vi "EventBuilder.ProcEvents.vi"(0 "i ref in":refnum<vi>, 5 "error in (no error)":errorcluster) -> (14 "i ref out":refnum<vi>, 19 "error out":errorcluster)   [LabVIEW 2014, in "EventBuilder.lvlib"]
doc: "This method is used to define the events the object will listen to. Add your own events here."
uses:
  EventBuilder.lvlib
  CSCore/BaseProcess/BaseProcess.event definition.ctl
  CSCore/CAEObj/CAEObj.event definition.ctl
  CSCore/BaseProcess/BaseProcess.descriptor string definition.ctl
  CSCore/BaseProcess/BaseProcess.lvlib
  CSCore/CAEObj/CAEObj.lvlib
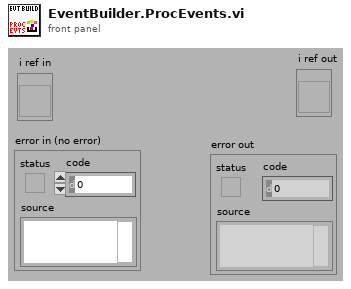
[diagram p1: front panel]
types:
  T1 = typedef "BaseProcess.lvlib/BaseProcess.event definition.ctl" = cluster{"CAEEvtDef":T2, "Data Descriptor":T3}
  T2 = typedef "CAEObj.lvlib/CAEObj.event definition.ctl" = cluster{"URL":string, "enable":bool, "ignoreResID":bool}
  T3 = typedef "BaseProcess.lvlib/BaseProcess.descriptor string definition.ctl" = string
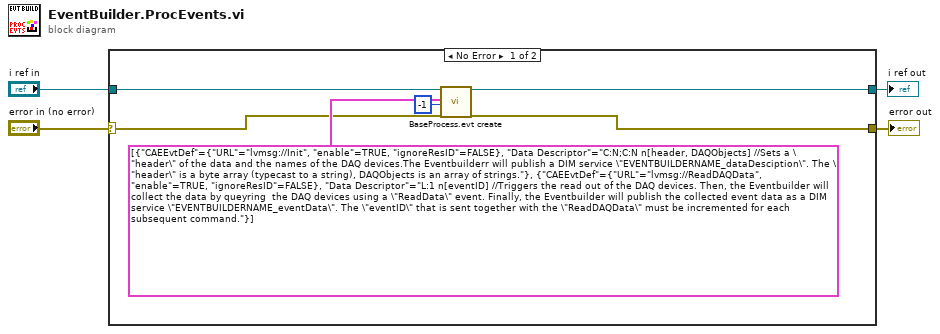
[diagram p0: block diagram]
diagram:
  n1 = case shown="No Error" "error in (no error)" {
    selector: "error in (no error)" -> [w6 w11]
    tunnel: "i ref in" -> [w10 w12]
    tunnel: [w9 w12] -> w3
    tunnel: [w8 w11] -> w2
    frame No Error {
      n2 = call "BaseProcess.evt create.vi"("i ref in"=w10, "newEvents"=T1[] [{"CAEEvtDef"={"URL"="lvmsg://Init", "enable"=TRUE, "ignoreResID"=FALSE}, "Data Descriptor"="C:N;C:N n[header, DAQObjects] //Sets a \"header\" of the data and the names of the DAQ devices.The Eventbuilderr will publish a DIM service \"EVENTBUILDERNAME_dataDesciption\". The \"header\" is a byte array (typecast to a string), DAQObjects is an array of strings."}, {"CAEEvtDef"={"URL"="lvmsg://ReadDAQData", "enable"=TRUE, "ignoreResID"=FALSE}, "Data Descriptor"="L:1 n[eventID] //Triggers the read out of the DAQ devices. Then, the Eventbuilder will collect the data by queyring  the DAQ devices using a \"ReadData\" event. Finally, the Eventbuilder will publish the collected event data as a DIM service \"EVENTBUILDERNAME_eventData\". The \"eventID\" that is sent together with the \"ReadDAQData\" must be incremented for each subsequent command."}] ("new events"), "ms timeout (10000)"=-1, "error in (no error)"=w6) -> ("i ref out"=w9:refnum<vi>, "error out"=w8:errorcluster)  [unwired: 12 in, 2 out]
    }
    frame Error {
    }
  }
  "i ref out" <- w3
  "error out" <- w2
